vi "GdsLanguage_GetTranslatedString.vi"(0 "StringID(s)":variant, 2 "GenerateErrorIfStringNotFoundInCURRENTLanguage (F)":bool, 5 "error in (no error)":errorcluster) -> (14 "FirstStringOut":string, 15 "SecondStringOut":string, 16 "StringsOut":string[](array[string]), 19 "error out":errorcluster)   [LabVIEW 2012]
doc: "Returns a translated string based on the value of the StringID parameter."
uses:
  <resource>/Framework/Providers/Open_GDS/SubVIs/GOOP_ErrorCodes.ctl
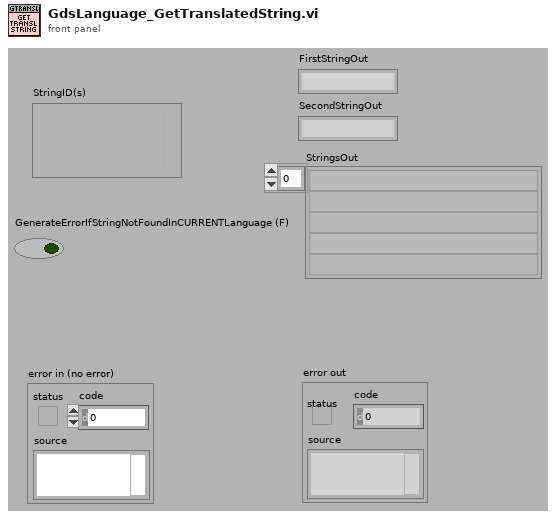
[diagram p1: front panel]
types:
  T1 = typedef "GOOP_ErrorCodes.ctl" = enum16{"LicenseFileMissing", "LicenseFileNotCorrect", "NoProductAccessGranted", "AgreementNoAccepted", "NoValidProviderFound", "LicenseExpired", "LanguageUndefined", "LanguageFileMissing", "LanguageFileChecksumError", "DublicateLanguageTranslation", "LanguageStringIDNotFound", "CommunityLimitReached", "ClassFileLocked", "ClassFileReadOnly", "ProjectNotValid"}
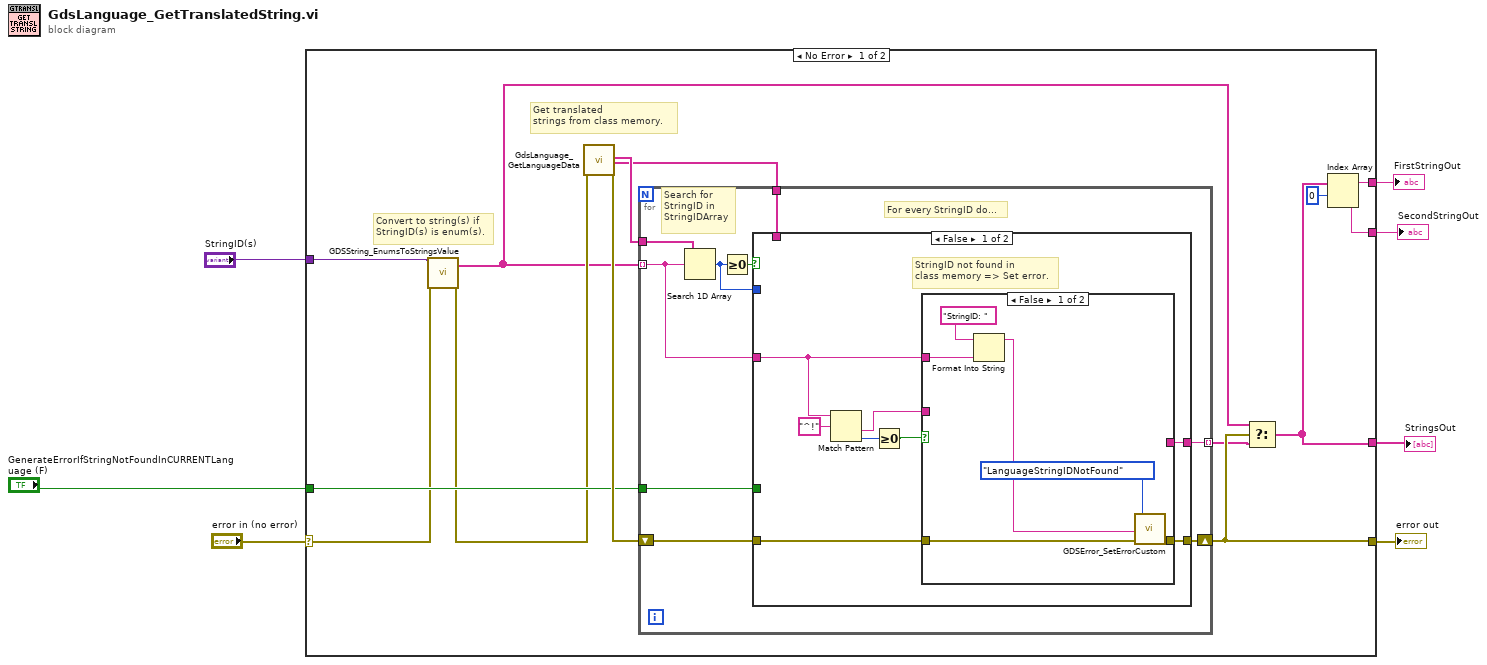
[diagram p0: block diagram]
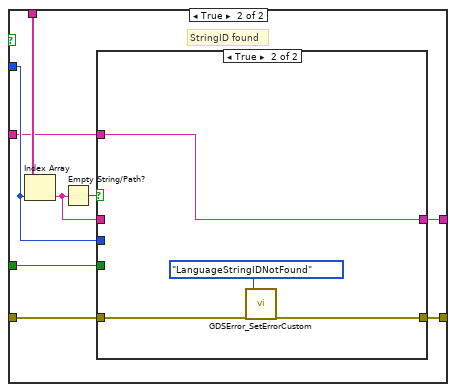
[diagram p3: hidden frame]
diagram:
  n1 = case shown="No Error" "error in (no error)" {
    selector: "error in (no error)" -> [w12 w62]
    tunnel: [w17 w62] -> w6
    tunnel: "StringID(s)" -> [w10 _]
    tunnel: [w21 _] -> w4
    tunnel: [w15 _] -> w3
    tunnel: "GenerateErrorIfStringNotFoundInCURRENTLanguage (F)" -> [w18 _]
    tunnel: [w8 _] -> w1
    frame No Error {
      # "Get translated\nstrings from class memory."
      # "Convert to string(s) if \nStringID(s) is enum(s)."
      n2 = call <resource>:"GDSString_EnumsToStringsValue.vi"("VariantIn(Enum(s) or String(s), could be an array)"=w10, "error in (no error)"=w12) -> ("StringsOut"=w9:string[], "error out"=w11:errorcluster)  [unwired: 15 in, 1 out]
      n3 = call <resource>:"GdsLanguage_GetLanguageData.vi"("error in (no error)"=w11) -> ("StringIDArray"=w14:string[], "TranslatedStrings"=w13:string[], "error out"=w19:errorcluster)  [unwired: 14 in, 2 out]
      n4 = for {
        tunnel: w9 -> [w22] mode=indexing
        tunnel: w14 -> [w30]
        tunnel: w13 -> [w29]
        tunnel: [w26] -> w16 mode=indexing
        shift-right: [w24] -> w17
        shift-left: w19 -> [w25]
        tunnel: w18 -> [w23]
        # "Search for\nStringID in \nStringIDArray"
        # "For every StringID do..."
        n5 = Search 1D Array(1D array=w30, element=w22) -> (index of element=w27:i32)  [unwired: 1 in]
        n6 = Greater Or Equal To 0?(x=w27) -> (x >= 0?=w28:bool)
        n7 = case shown="False" w28 {
          tunnel: w29 -> [_ w55]
          tunnel: w27 -> [_ w51]
          tunnel: [w32 w53] -> w26
          tunnel: w25 -> [w38 w49]
          tunnel: [w37 w50] -> w24
          tunnel: w23 -> [_ w48]
          tunnel: w22 -> [w36 w47]
          frame False {
            # "StringID not found in \nclass memory => Set error."
            n8 = Match Pattern(string=w36, regular expression="^!") -> (after substring=w31:string, offset past match=w34:i32)  [unwired: 1 in, 2 out]
            n9 = Greater Or Equal To 0?(x=w34) -> (x >= 0?=w33:bool)
            n10 = case shown="False" w33 {
              tunnel: w38 -> [w44 w46]
              tunnel: [w43 w46] -> w37
              tunnel: w36 -> [w40 _]
              tunnel: [_ w45] -> w32
              tunnel: w31 -> [_ w45]
              frame False {
                n11 = Format Into String(initial string="StringID: ", w40) -> (resulting string=w41:string)  [unwired: 2 in, 1 out]
                n12 = call <resource>:"GDSError_SetErrorCustom.vi"("source"=w41, "error in (no error)"=w44, "UserDefinedCodes(+5000)"=GOOP_ErrorCodes."LanguageStringIDNotFound") -> ("error out"=w43:errorcluster)  [unwired: 16 in]
              }
              frame True {
                # "BUT NOT IF THE FIRST\nCHARATER IS A !"
              }
            }
          }
          frame True {
            # "StringID found"
            n13 = Index Array(array=w55, index=w51) -> (element=w52:string)
            n14 = Empty String/Path?(string/path=w52) -> (empty?=w54:bool)
            n15 = case shown="True" w54 {
              tunnel: [w57 w58] -> w53
              tunnel: w52 -> [w57 _]
              tunnel: w51 -> [_ _]
              tunnel: [w56 w59] -> w50
              tunnel: w49 -> [w56 w60]
              tunnel: w48 -> [_ _]
              tunnel: w47 -> [_ w58]
              frame False {
                # "Translated string found for\ncurrent language => OK"
              }
              frame True {
                n16 = call <resource>:"GDSError_SetErrorCustom.vi"("error in (no error)"=w60, "UserDefinedCodes(+5000)"=GOOP_ErrorCodes."LanguageStringIDNotFound") -> ("error out"=w59:errorcluster)  [unwired: 17 in]
              }
            }
          }
        }
      }
      n17 = Select(t=w9, s=w17, f=w16) -> (s? t:f=w15:string[])
      n18 = Index Array(array=w15, index #1=0 ("index")) -> (element #1=w21:string, element #2=w8:string)  [unwired: 1 in]
    }
    frame Error {
    }
  }
  "error out" <- w6
  "FirstStringOut" <- w4
  "StringsOut" <- w3
  "SecondStringOut" <- w1
